vi "lib1.vi"() -> ()   [LabVIEW 2013]
panel:
  out "number":i32
  out "year of study":i32
  out "year":i32
  out "date string":string
  out "id number":i32
  out "offset string rollnumber":string
  out "Roll Number string":string
  out "Image Out":T1(plugin-control)
  in  "stop":bool
  # "Vision Acquision from ID Card"
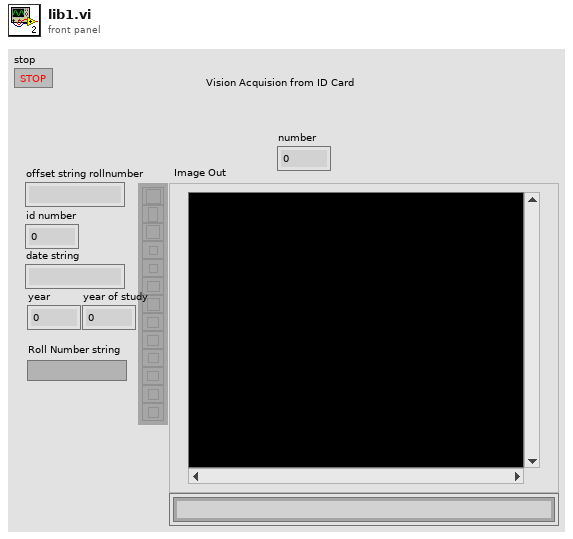
[diagram p1: front panel]
types:
  T1 = typedef "IMAQ Image.ctl" = refnum<image>
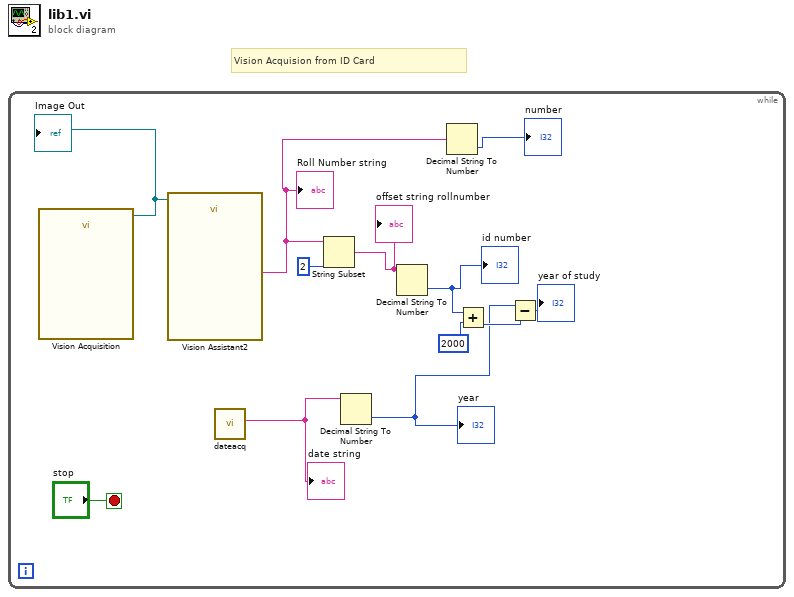
[diagram p0: block diagram]
diagram:
  # "Vision Acquision from ID Card"
  n1 = while {
    stop <- "stop" stop-if-true
    n2 = call "Vision Acquisition"() -> ("Image Out"=w12:T1)  [unwired: 24 in, 3 out]
    "Image Out" <- w12
    n3 = call "Vision Assistant2"("Image In"=w12) -> ("String (OCR/OCV 1)"=w1:string)  [unwired: 24 in, 2 out]
    "Roll Number string" <- w1
    n4 = call "dateacq.vi"() -> ("substring before match"=w3:string)  [unwired: 8 in, 3 out]
    "date string" <- w3
    n5 = String Subset(string=w1, length (rest)=2 ("length (rest)")) -> (substring=w9:string)  [unwired: 1 in]
    "offset string rollnumber" <- w9
    n6 = Decimal String To Number(string=w3) -> (number=w4:i32)  [unwired: 2 in, 1 out]
    "year" <- w4
    n7 = Decimal String To Number(string=w9) -> (number=w8:i32)  [unwired: 2 in, 1 out]
    "id number" <- w8
    n8 = Decimal String To Number(string=w1) -> (number=→"number":i32)  [unwired: 2 in, 1 out]
    n9 = Add(x=w8, y=2000) -> (x+y=w6:i32)
    n10 = Subtract(x=w4, y=w6) -> (x-y=→"year of study":i32)
  }
